vi "gen_laservoltage_sequence_scans.vi"(0 "V min":dbl, 5 "V max":dbl, 7 "# V steps":dbl, 11 "# Scans":i32) -> (6 "Voltage sequence":dbl[](array[numeric]), 10 "Total # data points":i32)   [LabVIEW 2012]
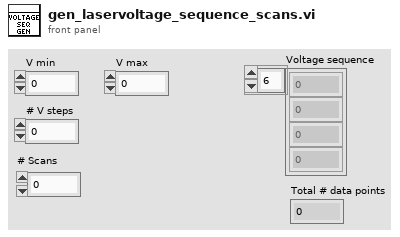
[diagram p1: front panel]
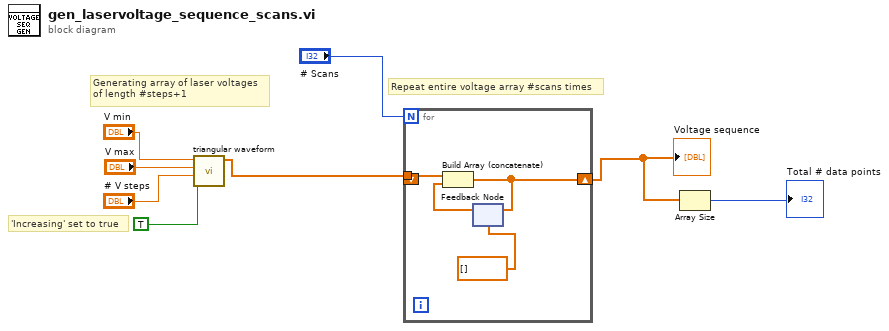
[diagram p0: block diagram]
diagram:
  # "Repeat entire voltage array #scans times"
  # "'Increasing' set to true"
  # "Generating array of laser voltages\nof length #steps+1"
  n1 = call "triangular waveform.vi"("Increasing?"=TRUE, "# of steps"="# V steps", "max"="V max", "min"="V min") -> ("data"=w2:dbl[])  [unwired: 7 in]
  n2 = for {
    N: "# Scans" -> [_]
    tunnel: w2 -> [w12]
    shift-right: [w9] -> w1
    shift-left: _ -> [_]
    n3 = feedback #1(dbl[] [] ("appended array")) -> (w11:dbl[])
    n4 = Build Array (concatenate)(w12, w11) -> (w9:dbl[])
    n5 = feedback-in #1(w9) -> ()
  }
  "Voltage sequence" <- w1
  n6 = Array Size(array=w1) -> (size(s)=→"Total # data points":i32)
